vi "_PI Receive String.vi"(0 "System no.":i32=1 min=1 step=1, 3 "Strip spaces?":bool, 5 "error in":errorcluster) -> (14 "String read":string, 15 "bytes read":u16, 19 "error out":errorcluster)   [LabVIEW 2014]
doc: "Read string from selected system.\n\nValid for all systems."
uses:
  _Available interfaces.ctl
  Public/PI/Mercury/GCS_LabVIEW/Low Level/Communication.llb/Available DLLs.ctl
  _Available DLL interfaces.ctl
  Public/PI/Mercury/GCS_LabVIEW/Low Level/Communication.llb/Termination character.ctl
  Public/PI/Mercury/GCS_LabVIEW/Low Level/Communication.llb/Global1.vi
panel:
  out "Logging mode":bool
  out "Syntax":enum16{"GCS 1.0", "GCS 2.0"}(ring)
  out "Termination character":T1
  out "VISA resource name":refnum<visa-resource-name>
  out "TCP/IP\nConfiguration":T2={"Host address/name"="localhost", "Port"=0, "Board"=4}
  out "DLL Interface Configuration":T5={"DLL for Device"=1, "DLL Interface"=0, "Parameter"=""} {"DLL Interface" items=["RS232", "GPIB", "Board", "TCP-IP", "USB", "RS232_DC"]; "DLL for Device" items=["C-843", "C-844", "E-710", "C-843.PM", "C-865", "E-761", "Mercury", "E-755", "E-753", "C-866", "E-712", "E-725", "E-861", "C-867", "E-517", "E-816"]}
  out "Interface configuration":T7={"RS232 Portnumber"=0, "Timeout"=5000, "RS232 baud rate"=57600, "Interface"=0, "GPIB Bus"=0, "GPIB address"=4, "GPIB Mode"=0} {"Interface" items=["RS232", "GPIB", "DLL", "TCP-IP", "USB", "Analog"]; "RS232 Portnumber" items=["COM1", "COM2", "COM3", "COM4", "COM5", "COM6", "COM7", "COM8", "COM9", "COM10", "COM11", "COM12", "COM13", "COM14", "COM15", "COM16", "COM17", "COM18", "COM19", "COM20", "COM21", "COM22", "COM23", "COM24", "COM25", "COM26", "COM27", "COM28", "COM29", "COM30"]}
  # "This vi receives a string via the selected interface."
  # "Communication setup indicators (for troubleshooting):"
  # "TCP/IP:"
  # "DLL:"
  # "General:"
  # "RS232:"
  # "GPIB:"
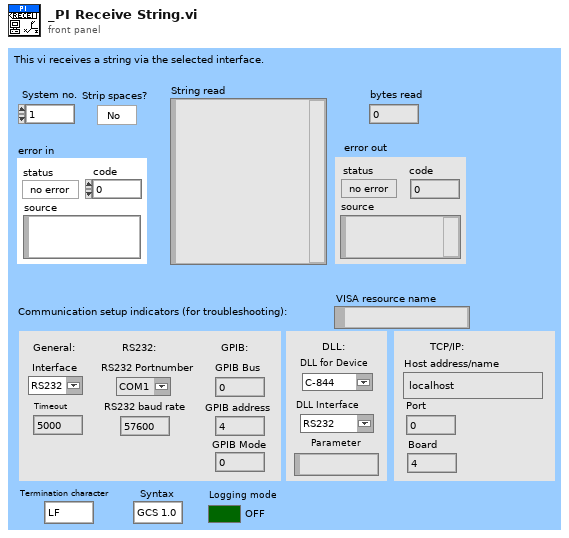
[diagram p1: front panel]
types:
  T1 = typedef "Termination character.ctl" = enum16{"LF", "CR", "LFCR", "CRLF"}
  T2 = cluster{"Host address/name":string, "Port":i32, "Board":i32}
  T3 = typedef "Available DLLs.ctl" = u16
  T4 = typedef "_Available DLL interfaces.ctl" = u16
  T5 = cluster{"DLL for Device":T3, "DLL Interface":T4, "Parameter":string}
  T6 = typedef "_Available interfaces.ctl" = u16
  T7 = cluster{"RS232 Portnumber":u16, "Timeout":u32, "RS232 baud rate":u32, "Interface":T6, "GPIB Bus":i16, "GPIB address":i16, "GPIB Mode":i16}
  T8 = typedef "Available DLL interfaces.ctl" = u16
  T9 = cluster{"DLL for Device":T3, "DLL Interface":T8, "Parameter":string}[]
  T10 = cluster{"Host address/name":string, "Port":i32, "Board":i32}[]
  T11 = typedef "Available interfaces.ctl" = u16
  T12 = cluster{"RS232 Portnumber":i32, "Timeout":i32, "RS232 Baud rate":u32, "Interface":T11, "GPIB Bus":i32, "GPIB Address":i32, "GPIB Mode":i32}[]
  T13 = cluster{"DLL for Device":T3, "DLL Interface":T8, "Parameter":string}
  T14 = cluster{"RS232 Portnumber":i32, "Timeout":i32, "RS232 Baud rate":u32, "Interface":T11, "GPIB Bus":i32, "GPIB Address":i32, "GPIB Mode":i32}
  T15 = enum16{"C844_IsDLLAvailable", "C844_ConnectRS232", "C844_ConnectNIgpib", "C844_IsConnected", "C844_CloseConnection", "C844_GcsCommandset", "C844_GetError", "C844_GcsGetAnswerSize", "C844_GcsGetAnswer", "C843_IsDLLAvailable", "C843_Connect", "C843_IsConnected", "C843_CloseConnection", "C843_GcsCommandset", "C843_GetError", "C843_GcsGetAnswerSize", "C843_GcsGetAnswer", "E710_IsDLLAvailable", "E710_ConnectRS232", "E710_ConnectNIgpib", "E710_IsConnected", "E710_CloseConnection", "E710_GcsCommandset", "E710_GetError", "E710_GcsGetAnswerSize", "E710_GcsGetAnswer", "C843_PM_IsDLLAvailable", "C843_PM_Connect", "C843_PM_IsConnected", "C843_PM_CloseConnection", "C843_PM_GcsCommandset", "C843_PM_GetError", "C843_PM_GcsGetAnswerSize", "C843_PM_GcsGetAnswer", "C843_PM_GetCurrentBoardID", "C843_GetCurrentBoardID", "C865_IsDLLAvailable", "C865_ConnectRS232", "C865_IsConnected", "C865_CloseConnection", "C865_GcsCommandset", "C865_GetError", "C865_GcsGetAnswerSize", "C865_GcsGetAnswer", "C865_GetCurrentInterfaceID", "E761_ConnectPciBoard", "DefineSystem", "CloseConnection", "IsConnected", "ConnectRS232", "ConnectNIgpib", "ConnectPciBoard", "ConnectTCPIP", "GetError", "GcsCommandset", "GCSGetAnswerSize", "GcsGetAnswer"}
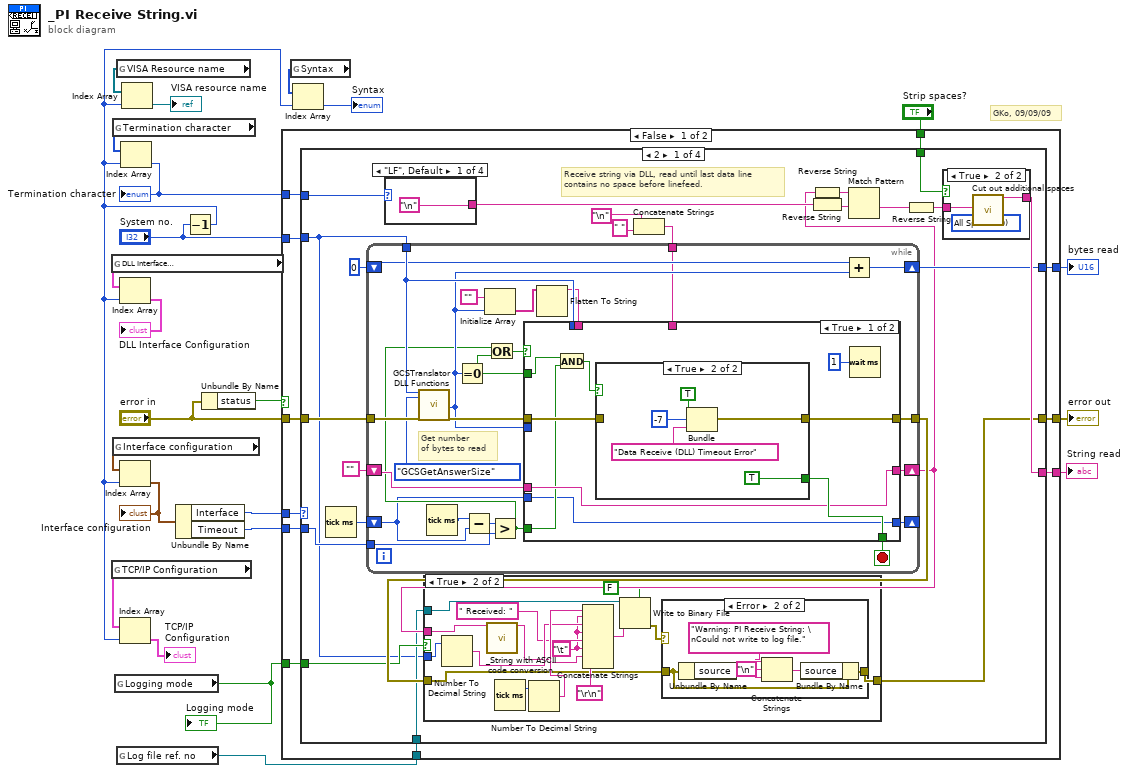
[diagram p0: block diagram]
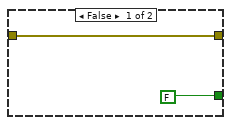
[diagram p4: hidden frame]
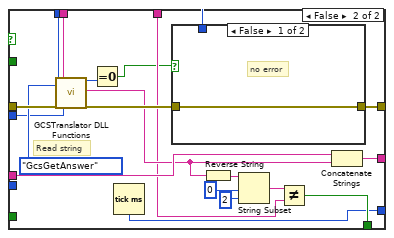
[diagram p5: hidden frame]
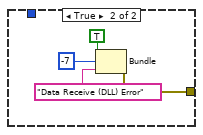
[diagram p6: hidden frame]
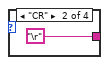
[diagram p7: hidden frame]
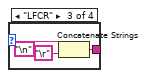
[diagram p8: hidden frame]
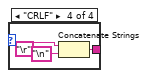
[diagram p9: hidden frame]
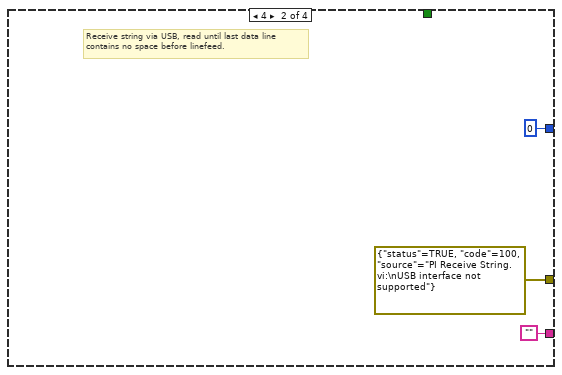
[diagram p11: hidden frame]
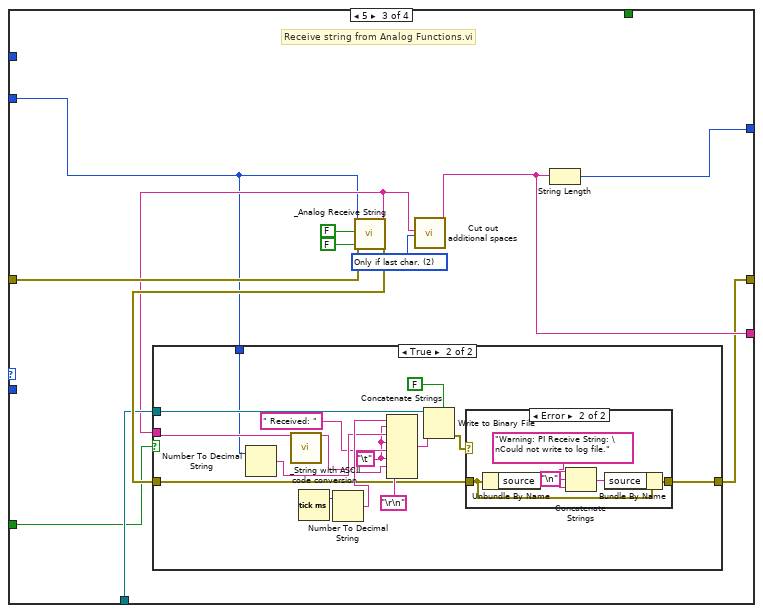
[diagram p12: hidden frame]
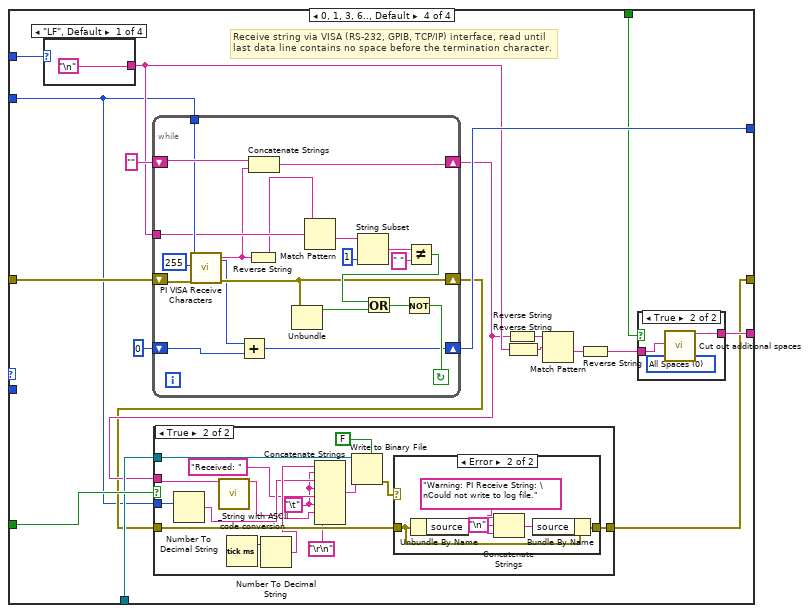
[diagram p15: hidden frame]
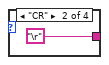
[diagram p19: hidden frame]
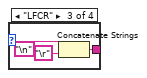
[diagram p20: hidden frame]
diagram:
  # "GKo, 09/09/09"
  n1 = global read "Global1.vi" "DLL Interface\nConfiguration"() -> (w16:T9)
  n2 = global read "Global1.vi" "TCP/IP Configuration"() -> (w11:T10)
  n3 = global read "Global1.vi" "Termination character"() -> (w9:T1[])
  n4 = global read "Global1.vi" "Interface configuration"() -> (w21:T12)
  n5 = global read "Global1.vi" "Logging mode"() -> (w2:bool)
  "Logging mode" <- w2
  n6 = global read "Global1.vi" "VISA Resource name"() -> (w13:refnum<visa-resource-name>[])
  n7 = global read "Global1.vi" "Log file ref. no"() -> (w1:refnum<file>)
  n8 = Decrement(x="System no.") -> (x-1=w3:i32)
  n9 = Index Array(array=w16, index=w3) -> (element=→"DLL Interface Configuration":T13)
  n10 = Index Array(array=w21, index=w3) -> (element=w14:T14)
  "Interface configuration" <- w14
  n11 = Index Array(array=w11, index=w3) -> (element=→"TCP/IP\nConfiguration":T2)
  n12 = Index Array(array=w9, index=w3) -> (element=w8:T1)
  "Termination character" <- w8
  n13 = Index Array(array=w13, index=w3) -> (element=→"VISA resource name":refnum<visa-resource-name>)
  n14 = Unbundle By Name(w14) -> ("Interface"=w17:T11, "Timeout"=w4:i32)
  n15 = Unbundle By Name("error in") -> ("status"=w18:bool)
  n16 = case shown="False" w18 {
    tunnel: [w35 "" ("String read")] -> w24
    tunnel: "error in" -> [w34 w268]
    tunnel: w17 -> [w33 _]
    tunnel: [w32 0 ("Bytes read")] -> w23
    tunnel: [w31 w268] -> w22
    tunnel: "System no." -> [w30 _]
    tunnel: w8 -> [w29 _]
    tunnel: "Strip spaces?" -> [w28 _]
    tunnel: w4 -> [w27 _]
    tunnel: w2 -> [w26 _]
    tunnel: w1 -> [w25 _]
    frame False {
      n17 = case shown="2" w33 {
        tunnel: [w57 "" ("String out") w169 w202] -> w35
        tunnel: w34 -> [w58 _ w166 w209]
        tunnel: [w49 0 w171 w210] -> w32
        tunnel: [w37 errorcluster {"status"=TRUE, "code"=100, "source"="PI Receive String.vi:\nUSB interface not supported"} w164 w196] -> w31
        tunnel: w30 -> [w36 _ w160 w195]
        tunnel: w29 -> [w52 _ _ w208]
        tunnel: w28 -> [w56 _ _ w201]
        tunnel: w27 -> [w42 _ _ _]
        tunnel: w26 -> [w39 _ w162 w200]
        tunnel: w25 -> [w38 _ w163 w199]
        frame 2 {
          # "Receive string via DLL, read until last data line\ncontains no space before linefeed."
          n18 = Tick Count (ms)() -> (millisecond timer value=w43:u32)
          n19 = case shown="\"LF\", Default" w52 {
            tunnel: ["\n" "\r" w147 w152] -> w51
            frame "LF", Default {
            }
            frame "CR" {
            }
            frame "LFCR" {
              n20 = Concatenate Strings("\n", "\r") -> (w147:string)
            }
            frame "CRLF" {
              n21 = Concatenate Strings("\r", "\n") -> (w152:string)
            }
          }
          n22 = Concatenate Strings("\n", " " ("string")) -> (w46:string)
          n23 = while {
            tunnel: w58 -> [w104]
            tunnel: [w103] -> w41
            tunnel: w36 -> [w102]
            shift-right: [w96] -> w49
            shift-left: 0 -> [w94]
            shift-right: [w93] -> w40
            shift-left: "" -> [w92]
            tunnel: w46 -> [w91]
            tunnel: w42 -> [w86]
            shift-right: [w83] -> _
            shift-left: w43 -> [w82]
            stop <- w90 stop-if-true
            # "Get number\nof bytes to read"
            n24 = call "GCSTranslator DLL Functions.vi"("System no."=w102, "Function"=T15."GCSGetAnswerSize", "error in"=w104) -> ("Numerical output"=w95:i32, "error out"=w98:errorcluster)  [unwired: 12 in, 3 out]
            n25 = Tick Count (ms)() -> (millisecond timer value=w88:u32)
            n26 = Equal To 0?(x=w95) -> (x = 0?=w84:bool)
            n27 = Subtract(x=w88, y=w82) -> (x-y=w87:u32)
            n28 = Initialize Array("", w95) -> (w100:string[])
            n29 = Greater?(x=w87, y=w86) -> (0:w85:bool)
            n30 = Or(x=w85, y=w84) -> (x .or. y?=w89:bool)
            n31 = Flatten To String(anything=w100) -> (data string=w99:string)  [unwired: 3 in, 2 out]
            n32 = case shown="True" w89 {
              tunnel: [w113 w139] -> w103
              tunnel: w102 -> [_ w138]
              tunnel: w99 -> [_ w137]
              tunnel: w98 -> [w112 w136]
              tunnel: w95 -> [_ w132]
              tunnel: [w109 w131] -> w93
              tunnel: w92 -> [w109 w130]
              tunnel: w91 -> [_ w125]
              tunnel: [w111 w124] -> w90
              tunnel: w85 -> [w108 _]
              tunnel: w84 -> [w107 _]
              tunnel: [w105 w121] -> w83
              tunnel: w82 -> [w105 _]
              frame True {
                n33 = And(x=w107, y=w108) -> (x .and. y?=w106:bool)
                n34 = case shown="True" w106 {
                  tunnel: [w115 w120] -> w113
                  tunnel: w112 -> [w115 _]
                  tunnel: [FALSE TRUE] -> w111
                  frame False {
                  }
                  frame True {
                    n35 = Bundle(TRUE, -7, "Data Receive (DLL) Timeout Error") -> (w120:errorcluster)  [unwired: 1 in]
                  }
                }
                n36 = Wait (ms)(milliseconds to wait=u32 1) -> ()  [unwired: 1 out]
              }
              frame False {
                # "Read string"
                n37 = call "GCSTranslator DLL Functions.vi"("System no."=w138, "Function"=T15."GcsGetAnswer", "error in"=w136, "String buffer"=w137, "Numerical input"=w132) -> ("DLL I32 Return value"=w135:i32, "String output"=w129:string, "error out"=w134:errorcluster)  [unwired: 10 in, 2 out]
                n38 = Equal To 0?(x=w135) -> (x = 0?=w122:bool)
                n39 = Tick Count (ms)() -> (millisecond timer value=w121:u32)
                n40 = case shown="False" w122 {
                  tunnel: [w140 w142] -> w139
                  tunnel: w138 -> [_ _]
                  tunnel: w134 -> [w140 _]
                  frame False {
                    # "no error"
                  }
                  frame True {
                    n41 = Bundle(TRUE, -7, "Data Receive (DLL) Error") -> (w142:errorcluster)  [unwired: 1 in]
                  }
                }
                n42 = Reverse String(1:w129) -> (0:w128:string)
                n43 = String Subset(string=w128, offset (0)=0, length (rest)=2 ("length (rest)")) -> (substring=w126:string)
                n44 = Not Equal?(x=w126, y=w125) -> (x != y?=w124:bool)
                n45 = Concatenate Strings(w130, w129) -> (w131:string)
              }
            }
            n46 = Add(x=w94, y=w95) -> (x+y=w96:i32)
          }
          n47 = case shown="True" w39 {
            tunnel: w38 -> [_ w63]
            tunnel: w40 -> [_ w62]
            tunnel: w41 -> [w59 w64]
            tunnel: [w59 w65] -> w37
            tunnel: w36 -> [_ w61]
            frame False {
            }
            frame True {
              w68 = "\t"
              n48 = Number To Decimal String(number=w61) -> (decimal integer string=w70:string)  [unwired: 1 in]
              n49 = call "_String with ASCII code conversion.vi"("Input string"=w62) -> ("Output string"=w67:string)  [unwired: 18 in]
              n50 = Tick Count (ms)() -> (millisecond timer value=w72:u32)
              n51 = Number To Decimal String(number=w72) -> (decimal integer string=w71:string)  [unwired: 1 in]
              n52 = Concatenate Strings(w71, w68, w70, w68, " Received: " ("string"), w68, w67, "\r\n") -> (w74:string)
              n53 = Write to Binary File(file (use dialog)=w63, data=w74, 5:FALSE ("prepend array or string size? (T)")) -> (error out=w73:errorcluster)  [unwired: 3 in, 2 out]
              n54 = case shown="Error" w73 {
                tunnel: w64 -> [w75 w81]
                tunnel: [w75 w77] -> w65
                frame No Error {
                }
                frame Error {
                  n55 = Unbundle By Name(w81) -> ("source"=w80:string)
                  n56 = Concatenate Strings(w80, "\n" ("string"), "Warning: PI Receive String: \nCould not write to log file." ("source")) -> (w76:string)
                  n57 = Bundle By Name(cluster=w81, "source"=w76) -> (w77:errorcluster)
                }
              }
            }
          }
          n58 = Reverse String(1:w40) -> (0:w54:string)
          n59 = Reverse String(1:w51) -> (0:w53:string)
          n60 = Match Pattern(string=w54, regular expression=w53) -> (after substring=w55:string)  [unwired: 1 in, 3 out]
          n61 = Reverse String(1:w55) -> (0:w50:string)
          n62 = case shown="True" w56 {
            tunnel: w50 -> [w153 w156]
            tunnel: [w153 w155] -> w57
            frame False {
            }
            frame True {
              w154 = u16 0 items=["All Spaces", "Only if 1st char.", "Only if last char.", "Only if near \"=\"", "Only if 1st or last char.", "Only multiple"] ("Mode")
              n63 = call "Cut out additional spaces.vi"("String"=w156, "Mode"=w154) -> ("String out"=w155:string)  [unwired: 17 in]
            }
          }
        }
        frame 4 {
          # "Receive string via USB, read until last data line\ncontains no space before linefeed."
        }
        frame 5 {
          w170 = u16 2 items=["All Spaces", "Only if 1st char.", "Only if last char.", "Only if near \"=\"", "Only if 1st or last char.", "Only multiple"] ("Mode")
          # "Receive string from Analog Functions.vi"
          n64 = call "_Analog Receive String.vi"("System no."=w160, "Read/Write (T)"=FALSE, "Ini"=FALSE, "error in"=w166) -> ("String out"=w161:string, "error out"=w165:errorcluster)  [unwired: 14 in]
          n65 = case shown="True" w162 {
            tunnel: w163 -> [_ w178]
            tunnel: w161 -> [_ w177]
            tunnel: w165 -> [w172 w176]
            tunnel: [w172 w175] -> w164
            tunnel: w160 -> [_ w174]
            frame False {
            }
            frame True {
              w181 = "\t"
              n66 = Number To Decimal String(number=w174) -> (decimal integer string=w183:string)  [unwired: 1 in]
              n67 = call "_String with ASCII code conversion.vi"("Input string"=w177) -> ("Output string"=w180:string)  [unwired: 18 in]
              n68 = Tick Count (ms)() -> (millisecond timer value=w185:u32)
              n69 = Number To Decimal String(number=w185) -> (decimal integer string=w184:string)  [unwired: 1 in]
              n70 = Concatenate Strings(w184, w181, w183, w181, " Received: " ("string"), w181, w180, "\r\n") -> (w187:string)
              n71 = Write to Binary File(file (use dialog)=w178, data=w187, 5:FALSE ("prepend array or string size? (T)")) -> (error out=w186:errorcluster)  [unwired: 3 in, 2 out]
              n72 = case shown="Error" w186 {
                tunnel: w176 -> [w188 w194]
                tunnel: [w188 w190] -> w175
                frame No Error {
                }
                frame Error {
                  n73 = Unbundle By Name(w194) -> ("source"=w193:string)
                  n74 = Concatenate Strings(w193, "\n" ("string"), "Warning: PI Receive String: \nCould not write to log file." ("source")) -> (w189:string)
                  n75 = Bundle By Name(cluster=w194, "source"=w189) -> (w190:errorcluster)
                }
              }
            }
          }
          n76 = call "Cut out additional spaces.vi"("String"=w161, "Mode"=w170) -> ("String out"=w169:string)  [unwired: 17 in]
          n77 = String Length(string=w169) -> (length=w171:i32)
        }
        frame 0, 1, 3, 6.., Default {
          # "Receive string via VISA (RS-232, GPIB, TCP/IP) interface, read until \nlast data line contains no space before the termination character."
          n78 = case shown="\"LF\", Default" w208 {
            tunnel: ["\n" "\r" w242 w247] -> w206
            frame "LF", Default {
            }
            frame "CR" {
            }
            frame "LFCR" {
              n79 = Concatenate Strings("\n", "\r") -> (w242:string)
            }
            frame "CRLF" {
              n80 = Concatenate Strings("\r", "\n") -> (w247:string)
            }
          }
          n81 = while {
            shift-left: w209 -> [w255]
            shift-right: [w254] -> w197
            tunnel: w195 -> [w253]
            shift-left: u16 0 -> [w260]
            shift-right: [w259] -> w210
            shift-left: "" -> [w267]
            shift-right: [w265] -> w198
            tunnel: w206 -> [w250]
            stop <- w262 continue-if-true
            n82 = call "PI VISA Receive Characters.vi"("System no."=w253, "Bytes to read"=u16 255, "error in"=w255) -> ("String read"=w248:string, "Bytes read"=w251:u16, "error out"=w254:errorcluster)  [unwired: 14 in]
            n83 = Add(x=w251, y=w260) -> (x+y=w259:u16)
            n84 = Reverse String(1:w248) -> (0:w249:string)
            n85 = Concatenate Strings(w267, w248) -> (w265:string)
            n86 = Unbundle(w254) -> ("status"=w264:bool)  [unwired: 2 out]
            n87 = Match Pattern(string=w249, regular expression=w250) -> (after substring=w256:string)  [unwired: 1 in, 3 out]
            n88 = String Subset(string=w256, length (rest)=1 ("length")) -> (substring=w257:string)  [unwired: 1 in]
            n89 = Not Equal?(x=w257, y=" ") -> (x != y?=w261:bool)
            n90 = Or(x=w261, y=w264) -> (x .or. y?=w263:bool)
            n91 = Not(x=w263) -> (.not. x?=w262:bool)
          }
          n92 = case shown="True" w200 {
            tunnel: w199 -> [_ w228]
            tunnel: w198 -> [_ w223]
            tunnel: w197 -> [w213 w225]
            tunnel: [w213 w224] -> w196
            tunnel: w195 -> [_ w222]
            frame False {
            }
            frame True {
              w217 = "\t"
              n93 = Number To Decimal String(number=w222) -> (decimal integer string=w219:string)  [unwired: 1 in]
              n94 = call "_String with ASCII code conversion.vi"("Input string"=w223) -> ("Output string"=w216:string)  [unwired: 18 in]
              n95 = Tick Count (ms)() -> (millisecond timer value=w221:u32)
              n96 = Number To Decimal String(number=w221) -> (decimal integer string=w220:string)  [unwired: 1 in]
              n97 = Concatenate Strings(w220, w217, w219, w217, "Received: " ("string"), w217, w216, "\r\n") -> (w227:string)
              n98 = Write to Binary File(file (use dialog)=w228, data=w227, 5:FALSE ("prepend array or string size? (T)")) -> (error out=w226:errorcluster)  [unwired: 3 in, 2 out]
              n99 = case shown="Error" w226 {
                tunnel: w225 -> [w229 w235]
                tunnel: [w229 w231] -> w224
                frame No Error {
                }
                frame Error {
                  n100 = Unbundle By Name(w235) -> ("source"=w234:string)
                  n101 = Concatenate Strings(w234, "\n" ("string"), "Warning: PI Receive String: \nCould not write to log file." ("source")) -> (w230:string)
                  n102 = Bundle By Name(cluster=w235, "source"=w230) -> (w231:errorcluster)
                }
              }
            }
          }
          n103 = Reverse String(1:w198) -> (0:w205:string)
          n104 = Reverse String(1:w206) -> (0:w204:string)
          n105 = Match Pattern(string=w205, regular expression=w204) -> (after substring=w207:string)  [unwired: 1 in, 3 out]
          n106 = Reverse String(1:w207) -> (0:w203:string)
          n107 = case shown="True" w201 {
            tunnel: w203 -> [w236 w239]
            tunnel: [w236 w238] -> w202
            frame False {
            }
            frame True {
              w237 = u16 0 items=["All Spaces", "Only if 1st char.", "Only if last char.", "Only if near \"=\"", "Only if 1st or last char.", "Only multiple"] ("Mode")
              n108 = call "Cut out additional spaces.vi"("String"=w239, "Mode"=w237) -> ("String out"=w238:string)  [unwired: 17 in]
            }
          }
        }
      }
    }
    frame True {
      # "Error!"
    }
  }
  "String read" <- w24
  "bytes read" <- w23
  "error out" <- w22
  n109 = global read "Global1.vi" "Syntax"() -> (w6:enum16{"GCS 1.0", "GCS 2.0"}[])
  n110 = Index Array(array=w6, index=w3) -> (element=→"Syntax":enum16{"GCS 1.0", "GCS 2.0"})
